vi "Core Actor (ROOT) - Dispatch Message to Child (Nested_Actor).vi"(8 "error in (no error)":errorcluster, 11 "Child_1_Class in":refnum<class "GUI_Class.lvclass">) -> (0 "error out":errorcluster, 3 "Child_1_Class out":refnum<class "GUI_Class.lvclass">)   [LabVIEW 2023, in "GUI_Actor.lvlib" / "GUI_Class.lvclass"]
uses:
  GUI_Class.lvclass
  GUI - Ctrl - Trigger Event Cluster.ctl
  Usr Ev/GUI - Ctrl - Enum - Events.ctl
  GUI_Class.lvclass/GUI_Class.ctl
  GUI_Class Messages/Core Actor - Send Actor Message Msg/Core Actor - Send Actor Message Msg.lvclass/Core Actor - Send Actor Message Msg.ctl
  <vilib>/ActorFramework/Message Enqueuer/Message Enqueuer.lvclass/Message Enqueuer.ctl
  <vilib>/ActorFramework/Message Enqueuer/Enqueue.vi
  GUI_Class Messages/Core Actor - Send Actor Message Msg/Core Actor - Send Actor Message Msg.lvclass
  C:/Program Files/National Instruments/LabVIEW 2023/vi.lib/ActorFramework/Message/Message.lvclass
  <vilib>/ActorFramework/Message Priority Queue/Priority Enqueue.vi
panel:
  out "Child Trigger Event Cluster":T1
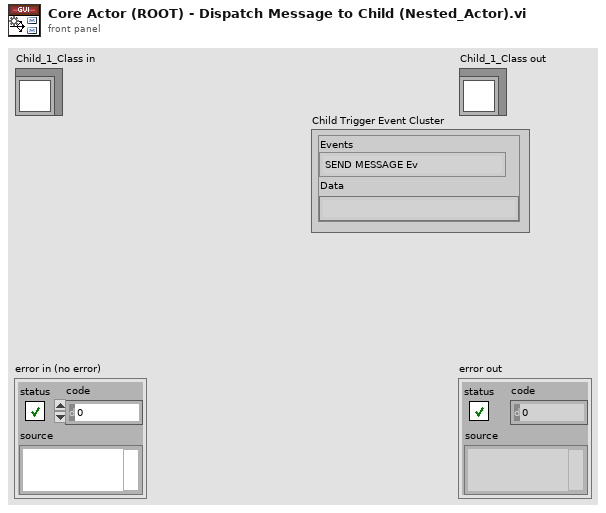
[diagram p1: front panel]
types:
  T1 = typedef "GUI_Actor.lvlib/GUI_Class.lvclass/GUI - Ctrl - Trigger Event Cluster.ctl" = cluster{"Events":T2, "Data":string}
  T2 = typedef "GUI_Actor.lvlib/GUI_Class.lvclass/GUI - Ctrl - Enum - Events.ctl" = enum16{"SEND MESSAGE Ev", "STOP_ACTOR Ev", "INIT_ACTOR Ev", "START Ev", "STOP Ev", "GET Ev", "SET Ev", "ERROR_HANDLER Ev", "RESET Ev", "T2 Ev", "T3 Ev", "T4 Ev"}
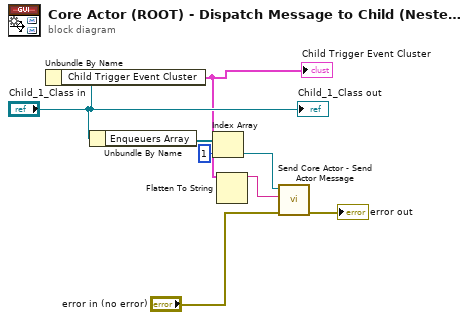
[diagram p0: block diagram]
diagram:
  n1 = Unbundle By Name("Child_1_Class in") -> ("Child Trigger Event Cluster"=w2:T1)
  "Child Trigger Event Cluster" <- w2
  n2 = Unbundle By Name("Child_1_Class in") -> ("Enqueuers Array"=w6:refnum<class "Message Enqueuer.lvclass">[])
  n3 = Index Array(array=w6, index=1) -> (element=w5:refnum<class "Message Enqueuer.lvclass">)
  n4 = Flatten To String(anything=w2) -> (data string=w1:string)  [unwired: 3 in, 2 out]
  n5 = call "Send Core Actor - Send Actor Message.vi"("error in (no error)"="error in (no error)", "Value"=w1, "Message Enqueuer"=w5) -> ("error out"=→"error out":errorcluster)  [unwired: 7 in, 1 out]
  "Child_1_Class out" <- "Child_1_Class in"
